vi "TALOS SVs path.vi"(8 "error in (no error)":errorcluster, 11 "Library Name":string) -> (0 "error out":errorcluster, 3 "Library path":path)   [LabVIEW 2020, in "TALOS.lvlib"]
uses:
  TALOS.lvlib
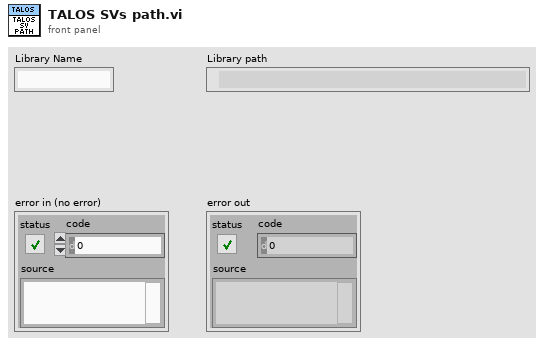
[diagram p1: front panel]
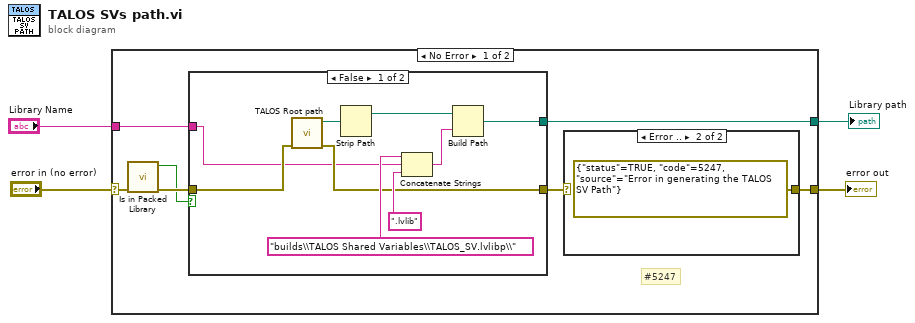
[diagram p0: block diagram]
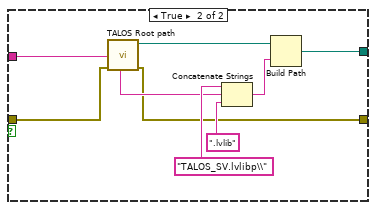
[diagram p3: hidden frame]
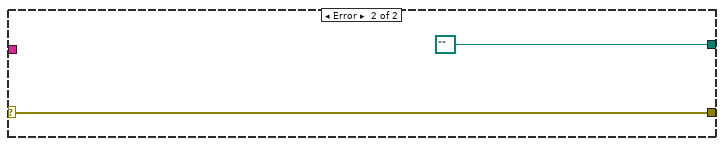
[diagram p4: hidden frame]
diagram:
  n1 = case shown="No Error" "error in (no error)" {
    selector: "error in (no error)" -> [w9 w32]
    tunnel: [w5 w32] -> w4
    tunnel: "Library Name" -> [w11 _]
    tunnel: [w10 path "" ("appended path")] -> w1
    frame No Error {
      # "#5247"
      n2 = call "Is in Packed Library.vi"("error in (no error)"=w9) -> ("error out"=w8:errorcluster, "Is In Packed Library"=w7:bool)  [unwired: 9 in]
      n3 = case shown="False" w7 {
        tunnel: [w18 w27] -> w10
        tunnel: w8 -> [w16 w26]
        tunnel: [w15 w23] -> w6
        tunnel: w11 -> [w14 w24]
        frame False {
          n4 = call "TALOS Root path.vi"("error in (no error)"=w16) -> ("error out"=w15:errorcluster, "TALOS Root Path"=w17:path)  [unwired: 9 in]
          n5 = Strip Path(path=w17) -> (stripped path=w20:path)  [unwired: 1 out]
          n6 = Concatenate Strings("builds\\TALOS Shared Variables\\TALOS_SV.lvlibp\\" ("string"), w14, ".lvlib" ("string")) -> (w19:string)
          n7 = Build Path(base path=w20, name or relative path=w19) -> (appended path=w18:path)
        }
        frame True {
          n8 = call "TALOS Root path.vi"("error in (no error)"=w26) -> ("error out"=w23:errorcluster, "TALOS Root Path"=w25:path)  [unwired: 9 in]
          n9 = Concatenate Strings("TALOS_SV.lvlibp\\" ("string"), w24, ".lvlib" ("string")) -> (w28:string)
          n10 = Build Path(base path=w25, name or relative path=w28) -> (appended path=w27:path)
        }
      }
      n11 = case shown="Error .." w6 {
        selector: w6 -> [w12 _]
        tunnel: [w12 errorcluster {"status"=TRUE, "code"=5247, "source"="Error in generating the TALOS SV Path"} ("error IO")] -> w5
        frame No Error {
        }
        frame Error {
        }
      }
    }
    frame Error {
    }
  }
  "error out" <- w4
  "Library path" <- w1
